vi "WLAN - QCA - UUT - AutoTest(Rx_PER).vi"(5 "VSG Resource Name":refnum<k15>="RIO0", 6 "Calibration Folder Path":path=path "C:/WLAN Reference/System Calibration", 8 "error in (no error)":errorcluster, 9 "NI HW":bool=TRUE, 10 "NART TCP Connection":refnum<k5>) -> (0 "error out":errorcluster, 3 "CART TCP Connection Out":refnum<k5>)   [LabVIEW 2011]
uses:
  <instrlib>/niRFSG/niRFSG.llb/niRFSG Ref Clock Sources.ctl
panel:
  in  "Tab Control":enum32{"HW "}(tab)
  out "Total Test Time (min)":dbl=0.7211833333332227
  # "GET PACKET COUNT (1)"
  # "PACKET STOP"
  # "PACKET START"
  # "GET PACKET COUNT (2)"
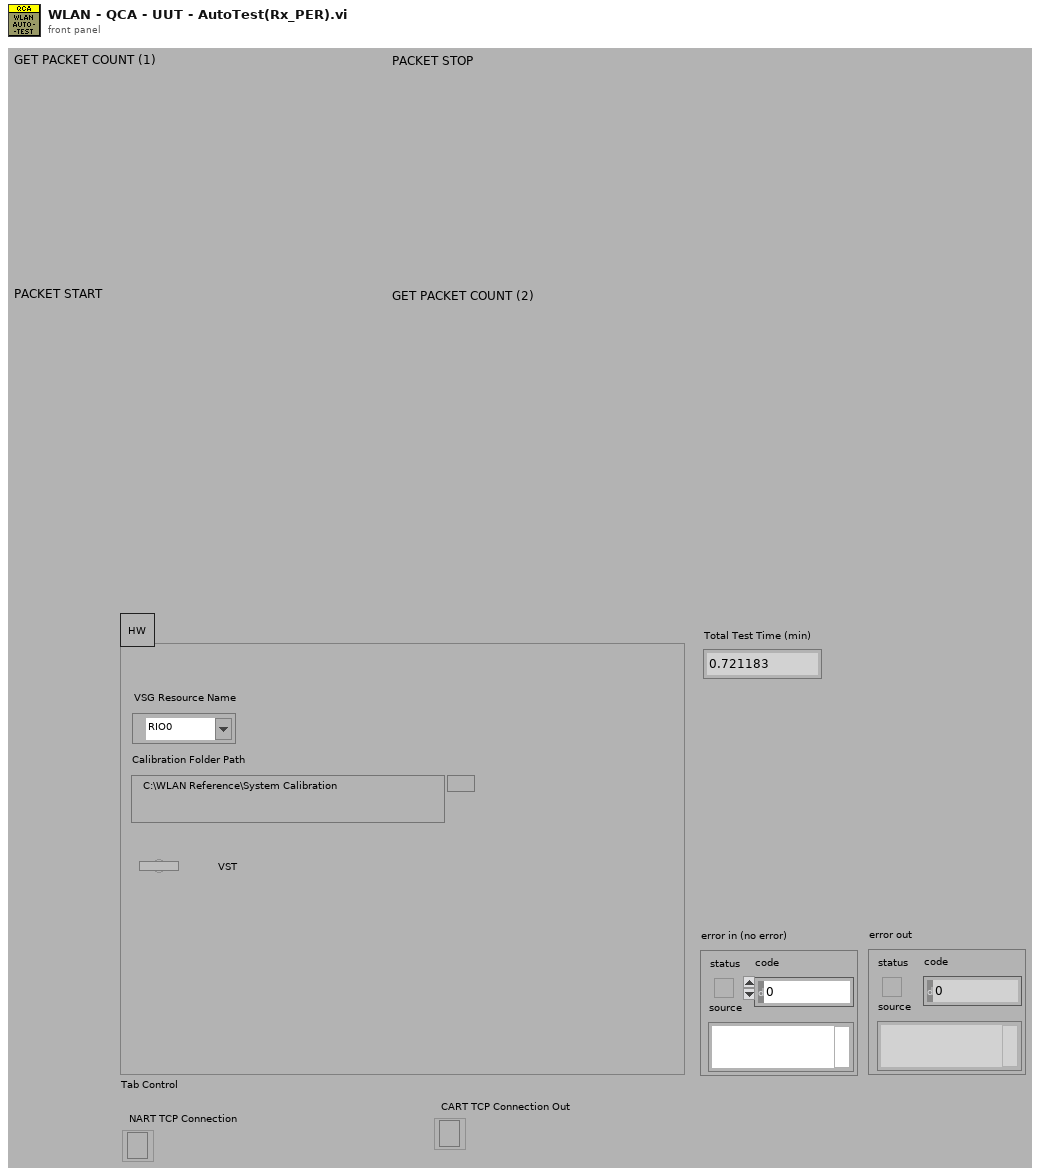
[diagram p1: front panel]
types:
  T1 = typedef "niRFSG Ref Clock Sources.ctl" = string
  T2 = typedef "WLAN - TV - RW - INC - Rx_PER_Sweep_Settings.ctl" = cluster{"Wfm_Index":i32, "Power Level Settings":cluster{"Stop Power Level(dBm)":dbl, "Start Power Level(dBm)":dbl, "Step Size":dbl}, "Carrier Frequency(Hz)":dbl, "# Freq Points":i32}
  T3 = typedef "WLAN - TV - RW - INC - Rx_PER_Wfm_Settings.ctl" = cluster{"Standard":i32, "Channel Bandwidth (Hz)":dbl, "Idle Interval (s)":dbl, "MCS Index":i32, "80211n PLCP Frame Format":i32, "Payload Data Length (bytes)":i32, "OFDM Data Rate (Mbps)":i32, "DSSS Data Rate (Mbps)":i32, "Wfm_Index":i32}
  T4 = cluster{"Temperature, C":dbl, "Time Stamp, sec":dbl, "Calibration Table":dbl[][]}
  T5 = typedef "WLAN - TV - RW - INC - RxTestParameters.ctl" = cluster{"wfm Size in msec":i32, "actual headroom (dB)":dbl, "Size in Samples":i32[], "40M?":bool, "Standard ":i32, "wfm size sec (dbl)":dbl, "dt":dbl, "Channel Bandwidth (Hz)":dbl, "Payload Data Length (bytes)":i32, "80211n PLCP Frame Format":i32, "DSSS Data Rate (Mbps)":i32, "OFDM Data Rate (Mbps)":i32, "MCS Index":i32, "Fc(Hz)":dbl, "#Packets":i32}
  T6 = typedef "Data Rates.ctl" = string
  T7 = cluster{"Frequency, MHz":u32, "Data Rate":T6, "Packet Count":i32, "RX Mac Address":string, "TX Mac Address":string, "BS Mac Address":string, "Packet Length":u32, "Broadcast":bool}
  T8 = cluster{"Correct Frames":i32, "Throughput":i32, "Error":i32}
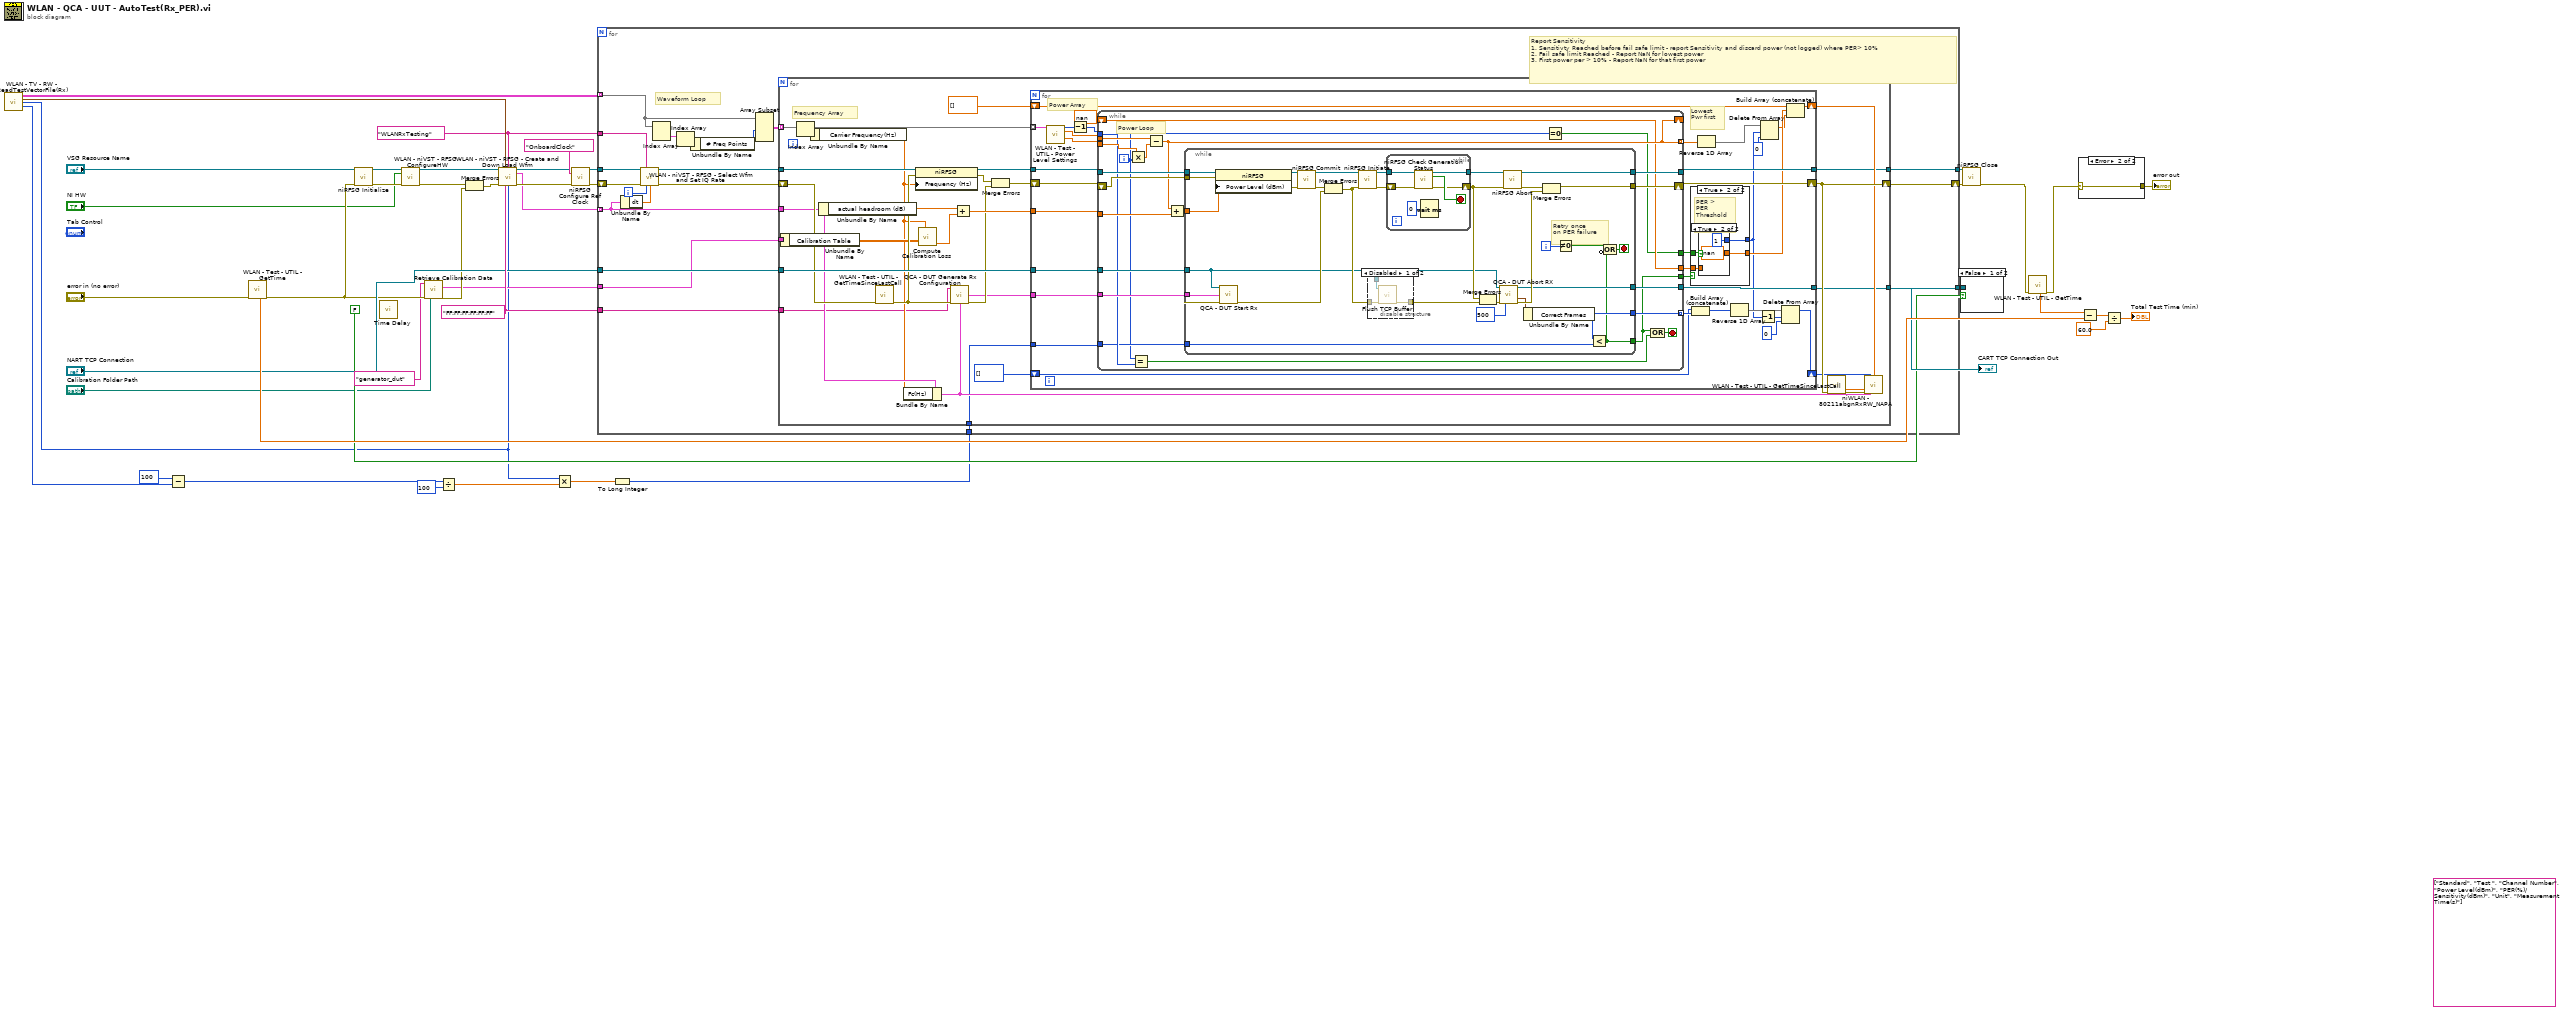
[diagram p0: block diagram]
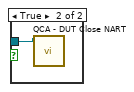
[diagram p2: hidden frame]
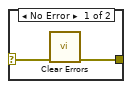
[diagram p3: hidden frame]
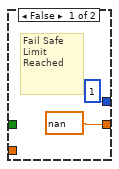
[diagram p4: hidden frame]
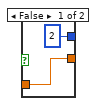
[diagram p5: hidden frame]
diagram:
  w20 = "FF:FF:FF:FF:FF:FF" ("Address String")
  w29 = "WLANRxTesting" ("Arb:Selected Script")
  (unwired) string[] ["Standard", "Test ", "Channel Number", "Power Level(dBm)", "PER(%)/Sensitivity(dBm)", "Unit", "Measurement Time(s)"]
  n1 = call "WLAN - TV - RW - ReadTestVectorFile(Rx).vi"() -> ("PER Sweep Settings(Wfm * FreQ * Pwr)"=w40:T2[][][], "Waveform Generation Settings"=w38:T3[], "#Packets"=w2:i32, "PER Threshold"=w1:i32)  [unwired: 12 in]
  n2 = Subtract(x=100, y=w1) -> (x-y=w7:i32)
  n3 = call "WLAN - Test - UTIL - GetTime.vi"("error in (no error)"="error in (no error)") -> ("error out"=w14:errorcluster, "Tick Count(s)"=w24:dbl)  [unwired: 8 in, 1 out]
  n4 = call <instrlib>:"niRFSG Initialize.vi"("resource name"="VSG Resource Name", "error in"=w14) -> ("instrument handle"=w19:refnum<k15>, "error out"=w39:errorcluster)  [unwired: 12 in]
  n5 = call "Time Delay"() -> ()  [unwired: 11 in, 1 out]
  n6 = call "WLAN - niVST - RFSG - ConfigureHW.vi"("instrument handle"=w19, "NI HW"="NI HW", "error in"=w39) -> ("instrument handle"=w37:refnum<k15>, "error out"=w31:errorcluster)  [unwired: 11 in]
  n7 = call "Retrieve Calibration Data.vi"("Calibration Signal Path Name"="generator_dut" ("Address String"), "error in (no error)"=w14, "Folder Path"="Calibration Folder Path") -> ("Calibration Data"=w10:T4, "error out"=w13:errorcluster)  [unwired: 11 in]
  n8 = Divide(x=w7, y=100) -> (x/y=w5:dbl)
  n9 = Merge Errors(w31, w13) -> (w30:errorcluster)
  n10 = call "WLAN - niVST - RFSG - Create and Down Load Wfm.vi"("instrument handle"=w37, "Waveform Generation Settings"=w38, "ScriptName<index>"=w29, "error in"=w30, "Address String"=w20, "numPackets"=w2) -> ("instrument handle"=w36:refnum<k15>, "Test Paramaters"=w34:T5[], "error out"=w35:errorcluster)  [unwired: 7 in]
  n11 = Multiply(x=w2, y=w5) -> (x*y=w6:dbl)
  n12 = call <instrlib>:"niRFSG Configure Ref Clock.vi"("instrument handle"=w36, "ref clock source"=T1 "OnboardClock", "error in"=w35) -> ("instrument handle out"=w33:refnum<k15>, "error out"=w32:errorcluster)  [unwired: 11 out]
  n13 = To Long Integer(number=w6) -> (32bit integer=w3:i32)
  n14 = for {
    tunnel: "NART TCP Connection" -> [w63]
    shift-right: [w64] -> w42
    shift-left: w32 -> [w53]
    tunnel: w33 -> [w54]
    tunnel: w34 -> [w51] mode=indexing
    tunnel: w40 -> [w61] mode=indexing
    tunnel: w29 -> [w52]
    tunnel: w20 -> [w49]
    tunnel: [w48] -> w18
    tunnel: [w47] -> w16
    tunnel: w10 -> [w46]
    tunnel: w3 -> [w45]
    i -> [w56]
    # "Report Sensitivity\n1. Sensitivty Reached before fail safe limit - report Sensitivity and discard power (not logged) where PER> 10%\n2. Fail safe limit Reached - Report NaN for lowest power\n3. First power per > 10% - Report NaN for that first power"
    # "Waveform Loop"
    n15 = Unbundle By Name(w51) -> ("dt"=w57:dbl)
    n16 = call "WLAN - niVST - RFSG - Select Wfm and Set IQ Rate.vi"("instrument handle"=w54, "Wfm Name"=w52, "error in"=w53, "Wfm Index"=w56, "dt"=w57) -> ("instrument handle"=w55:refnum<k15>, "error out"=w50:errorcluster)  [unwired: 9 in]
    n17 = Index Array(array=w61) -> (element=w60:T2[])  [unwired: 2 in]
    n18 = Index Array(array=w60) -> (element=w59:T2)  [unwired: 1 in]
    n19 = Unbundle By Name(w59) -> ("# Freq Points"=w58:i32)
    n20 = Array Subset(array=w61, length (row)=w58) -> (w62:T2[][])  [unwired: 3 in]
    n21 = for {
      tunnel: w63 -> [w91]
      shift-right: [w84] -> w64
      shift-left: w50 -> [w87]
      tunnel: w55 -> [w94]
      tunnel: w62 -> [w89] mode=indexing
      tunnel: w51 -> [w79]
      tunnel: w49 -> [w65]
      tunnel: [w72] -> w48
      tunnel: [w71] -> w47
      tunnel: w46 -> [w70]
      tunnel: w45 -> [w66]
      # "Frequency Array"
      n22 = Unbundle By Name(w70) -> ("Calibration Table"=w69:dbl[][])
      n23 = Index Array(array=w89) -> (element=w88:T2)  [unwired: 1 in]
      n24 = Unbundle By Name(w88) -> ("Carrier Frequency(Hz)"=w67:dbl)
      n25 = Unbundle By Name(w79) -> ("actual headroom (dB)"=w78:dbl)
      n26 = call "WLAN - Test - UTIL - GetTimeSinceLastCall.vi"("error in (no error)"=w87) -> ("error out"=w75:errorcluster)  [unwired: 9 in, 1 out]
      n27 = Bundle By Name(cluster=w79, "Fc(Hz)"=w67) -> (w73:T5)
      n28 = property class="niRFSG"(reference=w94, error in=w75, "Frequency (Hz)"=w67) -> (reference out=w93:refnum<k15>, error out=w92:errorcluster)
      n29 = call "Compute Calibration Loss.vi"("Table (frequency, power, pathloss)"=w69, "Center Frequency, Hz"=w67) -> ("External Attenuation, dB"=w68:dbl)  [unwired: 3 in, 2 out]
      n30 = call "QCA - DUT Generate Rx Configuration.vi"("Mac Address"=w65, "error in (no error)"=w75, "Rx_Test Parameters"=w73) -> ("Rx Configuration"=w74:T7, "error out"=w76:errorcluster)  [unwired: 10 in, 1 out]
      n31 = Add(x=w78, y=w68) -> (x+y=w77:dbl)
      n32 = Merge Errors(w92, w76) -> (w90:errorcluster)
      n33 = for {
        tunnel: w93 -> [w127]
        tunnel: w91 -> [w126]
        tunnel: w89 -> [w119] mode=indexing
        tunnel: w77 -> [w116]
        shift-right: [w124] -> w84
        shift-left: w90 -> [w125]
        shift-right: [w97] -> w81
        shift-left: i32[] [] -> [w121]
        shift-right: [w122] -> w80
        shift-left: dbl[] [] -> [w120]
        tunnel: w74 -> [w115]
        tunnel: [w114] -> w72
        tunnel: [w113] -> w71
        tunnel: w66 -> [w112]
        # "Lowest\nPwr first"
        # "Power Array"
        n34 = call "WLAN - Test - UTIL - Power Level Settings.vi"("Sweep Settings"=w119) -> ("# of Power Levels"=w111:i32, "Power Level Settings.Start Power Level(dBm)"=w117:dbl, "Power Level Settings.Step Size"=w118:dbl)  [unwired: 12 in]
        n35 = Decrement(x=w111) -> (x-1=w110:i32)
        n36 = while {
          tunnel: w126 -> [w150]
          shift-right: [w158] -> w124
          shift-left: w125 -> [w151]
          tunnel: w127 -> [w159]
          tunnel: [w145] -> w123 mode=indexing
          tunnel: w118 -> [w157]
          tunnel: w117 -> [w156]
          tunnel: w116 -> [w155]
          tunnel: [w143] -> w104 mode=indexing
          tunnel: w115 -> [w152]
          tunnel: [w149] -> w114
          tunnel: [w148] -> w113
          tunnel: w112 -> [w144]
          tunnel: w110 -> [w147]
          tunnel: [w139] -> w108
          shift-right: [w143] -> _
          shift-left: nan -> [w142]
          tunnel: [w142] -> w106
          tunnel: [w140] -> w107
          i -> [w141]
          stop <- w146 stop-if-true
          # "Power Loop"
          n37 = Multiply(x=w157, y=w141) -> (x*y=w153:dbl)
          n38 = Equal?(x=w141, y=w147) -> (x = y?=w138:bool)
          n39 = Subtract(x=w156, y=w153) -> (x-y=w143:dbl)
          n40 = Add(x=w143, y=w155) -> (x+y=w154:dbl)
          n41 = while {
            tunnel: w159 -> [w189]
            tunnel: [w187] -> w158
            tunnel: w154 -> [w180]
            tunnel: w152 -> [w179]
            tunnel: w151 -> [w178]
            tunnel: w150 -> [w170]
            tunnel: [w167] -> w149
            tunnel: [w166] -> w148
            tunnel: [w165] -> w145
            tunnel: w144 -> [w164]
            tunnel: [w160] -> w139
            i -> [w163]
            stop <- w161 stop-if-true
            # "Retry once\non PER failure"
            n42 = property class="niRFSG"(reference=w189, error in=w178, "Power Level (dBm)"=w180) -> (reference out=w184:refnum<k15>, error out=w181:errorcluster)
            n43 = call "QCA - DUT Start Rx.vi"("CART TCP Connection In"=w170, "Receive Config"=w179, "error in (no error)"=w178) -> ("error out"=w175:errorcluster)  [unwired: 10 in, 2 out]
            n44 = call <instrlib>:"niRFSG Commit.vi"("instrument handle"=w184, "error in"=w181) -> ("instrument handle out"=w183:refnum<k15>, "error out"=w174:errorcluster)  [unwired: 12 in]
            n45 = Merge Errors(w174, w175) -> (w176:errorcluster)
            n46 = call <instrlib>:"niRFSG Initiate.vi"("instrument handle"=w183, "error in"=w176) -> ("instrument handle out"=w186:refnum<k15>, "error out"=w182:errorcluster)  [unwired: 12 in]
            n47 = disable-structure shown="Disabled" {
              disable-tunnel: w176 -> [w192 w193]
              disable-tunnel: [w191 w193] -> w173
              disable-tunnel: w170 -> [w190 _]
              frame Disabled {
                n48 = call "Flush TCP Buffer.vi"("CART TCP Connection In"=w190, "error in (no error)"=w192) -> ("error out"=w191:errorcluster)  [unwired: 12 in, 1 out]
              }
              frame Enabled {
              }
            }
            n49 = while {
              tunnel: w186 -> [w199]
              tunnel: [w198] -> w185
              shift-right: [w196] -> w172
              shift-left: w182 -> [w195]
              stop <- w197 stop-if-true
              n50 = call <instrlib>:"niRFSG Check Generation Status.vi"("instrument handle"=w199, "error in"=w195) -> ("instrument handle out"=w198:refnum<k15>, "done?"=w197:bool, "error out"=w196:errorcluster)  [unwired: 11 in]
              n51 = Wait (ms)(milliseconds to wait=u32 0) -> ()  [unwired: 1 out]
            }
            n52 = Merge Errors(w172, w173) -> (w171:errorcluster)
            n53 = call "QCA - DUT Abort RX.vi"("CART TCP Connection In"=w170, "error in (no error)"=w171, "Read Time Out(ms)"=500) -> ("CART TCP Connection Out"=w166:refnum<k5>, "TX Response"=w168:T8, "error out"=w177:errorcluster)  [unwired: 10 in]
            n54 = call <instrlib>:"niRFSG Abort.vi"("instrument handle"=w185, "error in"=w172) -> ("instrument handle out"=w167:refnum<k15>, "error out"=w188:errorcluster)  [unwired: 12 in]
            n55 = Unbundle By Name(w168) -> ("Correct Frames"=w165:i32)
            n56 = Merge Errors(w188, w177) -> (w187:errorcluster)
            n57 = Not Equal To 0?(x=w163) -> (x != 0?=w162:bool)
            n58 = Less?(x=w165, y=w164) -> (x < y?=w160:bool)
            n59 = Compound Arithmetic op=OR(w162, invert w160) -> (w161:bool)
          }
          n60 = Equal To 0?(x=w141) -> (x = 0?=w140:bool)
          n61 = Compound Arithmetic op=OR(w139, w138) -> (w146:bool)
        }
        n62 = case shown="True" w108 {
          tunnel: w107 -> [_ w133]
          tunnel: w106 -> [_ w130]
          tunnel: [nan w131] -> w105
          tunnel: [1 ("length") w132] -> w96
          frame False {
            # "Fail Safe\nLimit\nReached"
          }
          frame True {
            # "PER >\nPER\nThreshold"
            n63 = case shown="True" w133 {
              tunnel: [2 ("length") 1 ("length")] -> w132
              tunnel: [w134 nan] -> w131
              tunnel: w130 -> [w134 _]
              frame False {
              }
              frame True {
              }
            }
          }
        }
        n64 = Build Array (concatenate)(w121, w123) -> (w100:i32[])
        n65 = Reverse 1D Array(array=w104) -> (reversed array=w103:dbl[])
        n66 = Reverse 1D Array(array=w100) -> (reversed array=w99:i32[])
        n67 = Decrement(x=w96) -> (x-1=w95:i32)
        n68 = Delete From Array(array=w103, length=w96, index=0 ("length")) -> (array with subset deleted=w101:dbl[])  [unwired: 1 out]
        n69 = Delete From Array(array=w99, length=w95, index=0 ("length")) -> (array with subset deleted=w97:i32[])  [unwired: 1 out]
        n70 = Build Array (concatenate)(w120, w105, w101) -> (w122:dbl[])
      }
      n71 = call "WLAN - Test - UTIL - GetTimeSinceLastCall.vi"("error in (no error)"=w84) -> ("error out"=w86:errorcluster, "Time Since Last Call (s)"=w85:dbl)  [unwired: 9 in]
      n72 = call "niWLAN - 80211abgnRxRW_NAPA.vi"("#Packets Received"=w81, "PowerLevel"=w80, "Test Time"=w85, "error in (no error)"=w86, "RxTestParameters"=w73) -> ()  [unwired: 11 in]
    }
  }
  "CART TCP Connection Out" <- w16
  n73 = case shown="False" FALSE {
    tunnel: w16 -> [_ w200]
    frame False {
    }
    frame True {
      n74 = call "QCA - DUT Close NART.vi"("CART TCP Connection"=w200) -> ()  [unwired: 14 in, 1 out]
    }
  }
  n75 = call <instrlib>:"niRFSG Close.vi"("instrument handle"=w18, "error in"=w42) -> ("error out"=w21:errorcluster)  [unwired: 13 in]
  n76 = call "WLAN - Test - UTIL - GetTime.vi"("error in (no error)"=w21) -> ("error out"=w27:errorcluster, "Tick Count(s)"=w25:dbl)  [unwired: 8 in, 1 out]
  n77 = case shown="Error" w27 {
    selector: w27 -> [w202 w203]
    tunnel: [w201 w203] -> w41
    frame No Error {
      n78 = call <vilib>:"Clear Errors.vi"("error in (no error)"=w202) -> ("error out"=w201:errorcluster)  [unwired: 6 in]
    }
    frame Error {
    }
  }
  "error out" <- w41
  n79 = Subtract(x=w25, y=w24) -> (x-y=w26:dbl)
  n80 = Divide(x=w26, y=60.0 ("x")) -> (x/y=→"Total Test Time (min)":dbl)
